vi "niFpga wdp fft 4-wire wrapper 2spc.vi"(0 "real data in":fxp<+/-,8,1>[](array[numeric])=[0.0, 0.0], 1 "reset":bool, 5 "imaginary data in":fxp<+/-,8,1>[](array[numeric])=[0.0, 0.0], 9 "input valid":bool, 12 "ready for output":bool) -> (3 "data indices":u16[](array[numeric]), 4 "real data out":fxp<+/-,19,12>[](array[numeric]), 6 "imaginary data out":fxp<+/-,19,12>[](array[numeric]), 10 "output valid":bool, 14 "ready for input":bool)   [LabVIEW 2017]
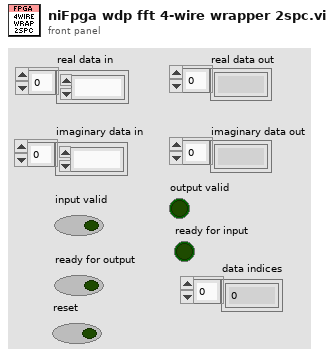
[diagram p1: front panel]
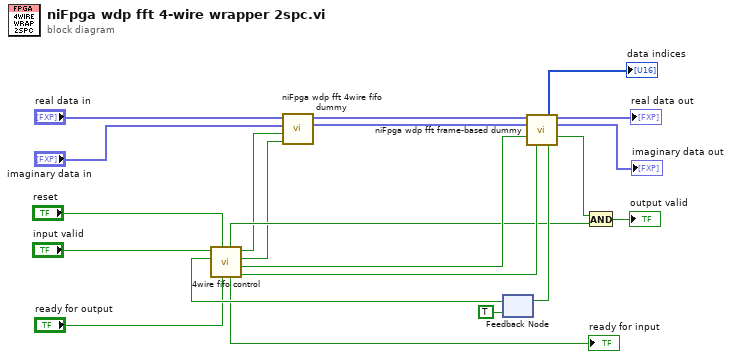
[diagram p0: block diagram]
diagram:
  n1 = feedback #1(TRUE ("ready for frame")) -> (w8:bool)
  n2 = call "4wire fifo control"("ready for output"="ready for output", "reset"="reset", "ready for frame"=w8, "input valid"="input valid") -> ("enable"=w5:bool, "frame start"=w4:bool, "read?"=w1:bool, "write?"=w2:bool, "ready for input"=→"ready for input":bool, "not in reset?"=w3:bool)  [unwired: 2 in]
  n3 = call <vilib>:"niFpga wdp fft 4wire fifo dummy.vi"("read?"=w1, "write?"=w2, "data in im"="imaginary data in", "data in re"="real data in") -> ("data out im"=w11:fxp<+/-,8,1>[], "data out re"=w13:fxp<+/-,8,1>[])  [unwired: 6 in]
  n4 = call <vilib>:"niFpga wdp fft frame-based dummy.vi"("real data in"=w13, "imaginary data in"=w11, "input frame start"=w4, "enable"=w5) -> ("data indices"=→"data indices":u16[], "real data out"=→"real data out":fxp<+/-,19,12>[], "imaginary data out"=→"imaginary data out":fxp<+/-,19,12>[], "output valid"=w16:bool, "ready for frame"=w18:bool)  [unwired: 6 in, 1 out]
  n5 = feedback-in #1(w18) -> ()
  n6 = And(x=w16, y=w3) -> (x .and. y?=→"output valid":bool)
